vi "rotm_siso.vi"(6 "angle[rad]":dbl, 7 "reverse":bool, 8 "y0":dbl, 9 "x0":dbl, 10 "y":dbl, 11 "x":dbl) -> (2 "y'":dbl, 3 "x'":dbl)   [LabVIEW 2015]
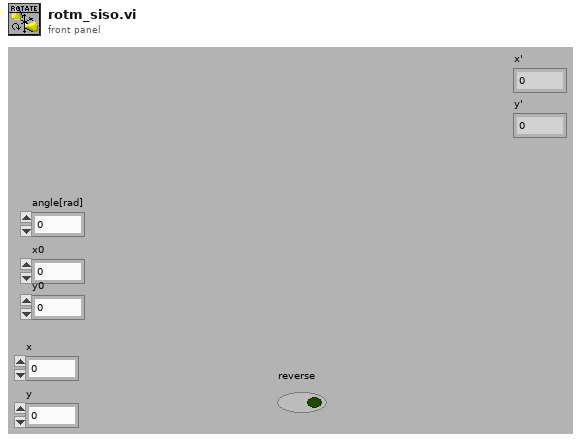
[diagram p1: front panel]
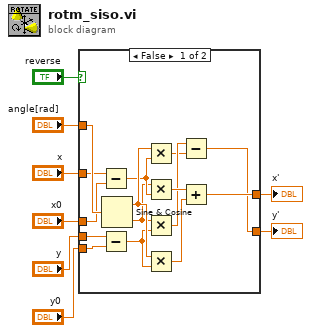
[diagram p0: block diagram]
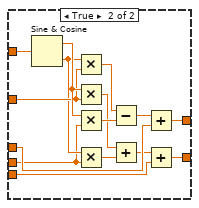
[diagram p2: hidden frame]
diagram:
  n1 = case shown="False" "reverse" {
    tunnel: "angle[rad]" -> [w23 w38]
    tunnel: "x" -> [w22 w31]
    tunnel: "x0" -> [w21 w34]
    tunnel: "y0" -> [w20 w25]
    tunnel: "y" -> [w19 w29]
    tunnel: [w16 w33] -> w2
    tunnel: [w9 w24] -> w1
    frame False {
      n2 = Subtract(x=w22, y=w21) -> (x-y=w14:dbl)
      n3 = Subtract(x=w19, y=w20) -> (x-y=w12:dbl)
      n4 = Sine & Cosine(0:w23) -> (1:w15:dbl, 2:w13:dbl)
      n5 = Multiply(x=w15, y=w14) -> (x*y=w10:dbl)
      n6 = Multiply(x=w13, y=w14) -> (x*y=w18:dbl)
      n7 = Multiply(x=w13, y=w12) -> (x*y=w11:dbl)
      n8 = Multiply(x=w15, y=w12) -> (x*y=w17:dbl)
      n9 = Subtract(x=w11, y=w10) -> (x-y=w9:dbl)
      n10 = Add(x=w18, y=w17) -> (x+y=w16:dbl)
    }
    frame True {
      n11 = Sine & Cosine(0:w38) -> (1:w32:dbl, 2:w30:dbl)
      n12 = Multiply(x=w30, y=w31) -> (x*y=w37:dbl)
      n13 = Multiply(x=w32, y=w31) -> (x*y=w28:dbl)
      n14 = Multiply(x=w32, y=w29) -> (x*y=w36:dbl)
      n15 = Multiply(x=w30, y=w29) -> (x*y=w27:dbl)
      n16 = Subtract(x=w37, y=w36) -> (x-y=w35:dbl)
      n17 = Add(x=w28, y=w27) -> (x+y=w26:dbl)
      n18 = Add(x=w35, y=w34) -> (x+y=w33:dbl)
      n19 = Add(x=w26, y=w25) -> (x+y=w24:dbl)
    }
  }
  "x'" <- w2
  "y'" <- w1
